vi "Audio Device Info.vi"(6 "isInput?":bool, 7 "device":u32, 8 "error in (no error)":errorcluster) -> (0 "error out":errorcluster, 4 "Capabilities":T1, 5 "Device Name":string)   [LabVIEW 2020]
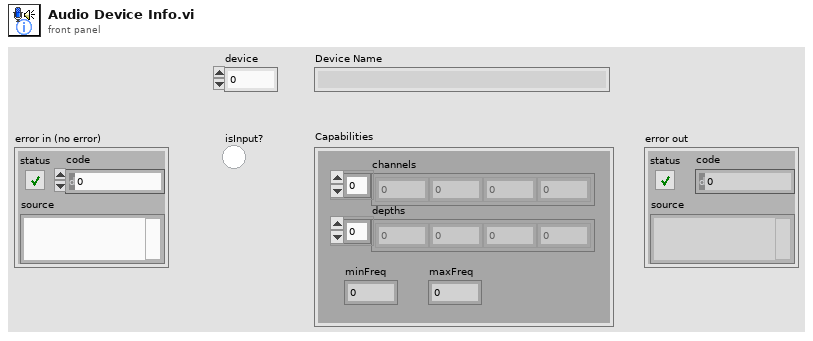
[diagram p1: front panel]
types:
  T1 = cluster{"channels":i32[], "depths":i32[], "minFreq":dbl, "maxFreq":dbl}
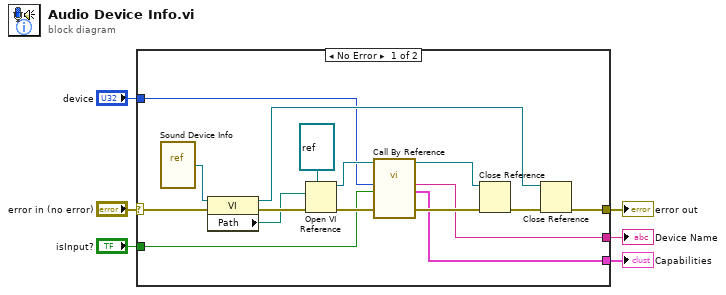
[diagram p0: block diagram]
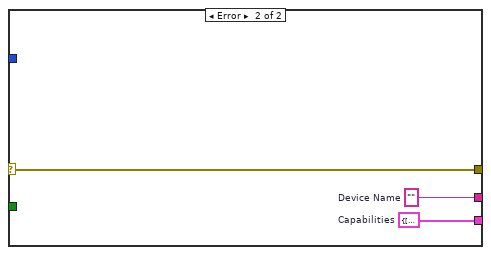
[diagram p2: hidden frame]
diagram:
  n1 = case shown="No Error" "error in (no error)" {
    selector: "error in (no error)" -> [w22 w25]
    tunnel: [w10 w24] -> w6
    tunnel: [w13 w25] -> w4
    tunnel: [w15 w23] -> w3
    tunnel: "device" -> [w9 _]
    tunnel: "isInput?" -> [w8 _]
    frame No Error {
      n2 = vi-ref <vilib>:"Sound Device Info.vi"() -> (w18:refnum<vi>)
      n3 = property class="VI"(reference=w18, error in=w22) -> (reference out=w12:refnum<vi>, error out=w21:errorcluster, "Path"=w19:path)
      n4 = Open VI Reference(type specifier VI Refnum (for type only)=refnum<vi> refnum, vi path=w19, error in (no error)=w21) -> (vi reference=w11:refnum<vi>, error out=w20:errorcluster)  [unwired: 3 in]
      n5 = call-by-ref "?"(reference=w11, "device"=w9, "isInput?"=w8, "error in (no error)"=w20) -> (reference out=w7:refnum<vi>, "Device Name"=w10:string, "Capabilities"=w15:T1, "error out"=w16:errorcluster)  [unwired: 11 in, 1 out]
      n6 = Close Reference(reference=w7, error in (no error)=w16) -> (error out=w14:errorcluster)
      n7 = Close Reference(reference=w12, error in (no error)=w14) -> (error out=w13:errorcluster)
    }
    frame Error {
      w23 = T1 {"channels"=[], "depths"=[], "minFreq"=0.0, "maxFreq"=0.0}  # Capabilities
      w24 = ""  # Device Name
    }
  }
  "Device Name" <- w6
  "error out" <- w4
  "Capabilities" <- w3
